vi "rsscope_core_global.vi"() -> ()   [LabVIEW 2014] (continued)
WfmRNOHist2, WfmTNTrack2, WfmDDNTrack2, WfmPNTrack2, WfmRNTrack2, WfmTNSpectrum2, WfmDDNSpectrum2, WfmPNSpectrum2, WfmRNSpectrum2, WfmPJDHist1, WfmBUJHist1, WfmRJHist1, WfmPJDTrack1, WfmPJDSpectrum1, WfmPJDHist2, WfmBUJHist2, WfmRJHist2, WfmPJDTrack2, WfmPJDSpectrum2, WfmPNDHist1, WfmBUNHist1, WfmRNHist1, WfmPNDTrack1, WfmPNDSpectrum1, WfmPNDHist2, WfmBUNHist2, WfmRNHist2, WfmPNDTrack2, WfmPNDSpectrum2\r\n\nRemote-control command(s):\nREFLevel<m>:AUTO:MODE"}, {"Level"=2, "Class Only"=FALSE, "Identifier"="RSSCOPE_ATTR_REFERENCE_LEVEL_AVERAGING_ENABLED", "Descriptive Name"="Reference Level Averaging Enabled", "Data Type"=3, "Command"="REFL{WfmSuffix}:AUTO", "Access"=2, "Range Table"="", "Read Callback"="", "Write Callback"="", "Supported Models"="", "Instrument Options"="", "Flags"=0, "Help"="Enables averaging over several histograms to determine the reference levels.\n\nAvailable Repeated Capabilities:\nWfmSuffix: WfmNone, WfmC1W1, WfmC1W2, WfmC1W3, WfmC2W1, WfmC2W2, WfmC2W3, WfmC3W1, WfmC3W2, WfmC3W3, WfmC4W1, WfmC4W2, WfmC4W3, WfmMath1, WfmMath2, WfmMath3, WfmMath4, WfmRef1, WfmRef2, WfmRef3, WfmRef4, WfmXY1, WfmXY2, WfmXY3, WfmXY4, WfmMeas1, WfmMeas2, WfmMeas3, WfmMeas4, WfmMeas5, WfmMeas6, WfmMeas7, WfmMeas8, WfmSbus1, WfmSbus2, WfmSbus3, WfmSbus4, WfmD0, WfmD1, WfmD2, WfmD3, WfmD4, WfmD5, WfmD6, WfmD7, WfmD8, WfmD9, WfmD10, WfmD11, WfmD12, WfmD13, WfmD14, WfmD15, WfmMSO1, WfmMSO2, WfmMSO3, WfmMSO4, WfmTRK1, WfmTRK2, WfmTRK3, WfmTRK4, WfmTRK5, WfmTRK6, WfmTRK7, WfmTRK8, WfmSpectrum1, WfmSpectrum2, WfmSpectrum3, WfmSpectrum4, WfmSG1TL1, WfmSG1TL2, WfmSG2TL1, WfmSG2TL2, WfmSG3TL1, WfmSG3TL2, WfmSG4TL1, WfmSG4TL2, WfmEye1, WfmEye2, WfmEye3, WfmEye4, WfmZ1V1, WfmZ1V2, WfmZ1V3, WfmZ1V4, WfmZ1I1, WfmZ1I2, WfmZ1I3, WfmZ1I4, WfmZ2V1, WfmZ2V2, WfmZ2V3, WfmZ2V4, WfmZ2I1, WfmZ2I2, WfmZ2I3, WfmZ2I4, WfmDiff1, WfmDiff2, WfmCommon1, WfmCommon2, WfmTDRZ, WfmTDRH, WfmTDRR, WfmMath5, WfmMath6, WfmMath7, WfmMath8, WfmSpectrum5, WfmSpectrum6, WfmSpectrum7, WfmSpectrum8, WfmSG5TL1, WfmSG5TL2, WfmSG6TL1, WfmSG6TL2, WfmSG7TL1, WfmSG7TL2, WfmSG8TL1, WfmSG8TL2, WfmHP1, WfmHP2, WfmHP3, WfmHP4, WfmHP5, WfmHP6, WfmHP7, WfmHP8, WfmHP9, WfmHP10, WfmBathtub1, WfmBathMeas1, WfmStepResp1, WfmSRHist1, WfmSDHist1, WfmTJHist1, WfmDJHist1, WfmDDJHist1, WfmPJHist1, WfmRJOHist1, WfmSRTrack1, WfmTJTrack1, WfmDJTrack1, WfmDDJTrack1, WfmPJTrack1, WfmRJTrack1, WfmTJSpectrum1, WfmDDJSpectrum1, WfmPJSpectrum1, WfmRJSpectrum1, WfmSEye1, WfmBathtub2, WfmBathMeas2, WfmStepResp2, WfmSRHist2, WfmSDHist2, WfmTJHist2, WfmDJHist2, WfmDDJHist2, WfmPJHist2, WfmRJOHist2, WfmSRTrack2, WfmSDTrack2, WfmTJTrack2, WfmDDJTrack2, WfmPJTrack2, WfmRJTrack2, WfmTJSpectrum2, WfmDDJSpectrum2, WfmPJSpectrum2, WfmRJSpectrum2, WfmSEye2, WfmNBathtub1, WfmNBathMeas1, WfmTNHist1, WfmDNHist1, WfmDDNHist1, WfmPNHist1, WfmRNOTrack1, WfmTNTrack1, WfmDDNTrack1, WfmPNTrack1, WfmRNTrack1, WfmTNSpectrum1, WfmDDNSpectrum1, WfmPNSpectrum1, WfmRNSpectrum1, WfmNBathtub2, WfmNBathMeas2, WfmTNHist2, WfmDNHist2, WfmDDNHist2, WfmPNHist2, WfmRNOHist2, WfmTNTrack2, WfmDDNTrack2, WfmPNTrack2, WfmRNTrack2, WfmTNSpectrum2, WfmDDNSpectrum2, WfmPNSpectrum2, WfmRNSpectrum2, WfmPJDHist1, WfmBUJHist1, WfmRJHist1, WfmPJDTrack1, WfmPJDSpectrum1, WfmPJDHist2, WfmBUJHist2, WfmRJHist2, WfmPJDTrack2, WfmPJDSpectrum2, WfmPNDHist1, WfmBUNHist1, WfmRNHist1, WfmPNDTrack1, WfmPNDSpectrum1, WfmPNDHist2, WfmBUNHist2, WfmRNHist2, WfmPNDTrack2, WfmPNDSpectrum2\r\n\nRemote-control command(s):\nREFLevel<m>:AUTO[:STATe]"}, {"Level"=2, "Class Only"=FALSE, "Identifier"="RSSCOPE_ATTR_REFERENCE_LEVEL_AVERAGING_COUNT", "Descriptive Name"="Reference Level Averaging Count", "Data Type"=0, "Command"="REFL{WfmSuffix}:AUTO:COUN", "Access"=2, "Range Table"="rsscope_rngRefLevelAvgCount", "Read Callback"="", "Write Callback"="", "Supported Models"="", "Instrument Options"="", "Flags"=0, "Help"="Defines the number of histograms to calculate the average from.\n\nAvailable Repeated Capabilities:\nWfmSuffix: WfmNone, WfmC1W1, WfmC1W2, WfmC1W3, WfmC2W1, WfmC2W2, WfmC2W3, WfmC3W1, WfmC3W2, WfmC3W3, WfmC4W1, WfmC4W2, WfmC4W3, WfmMath1, WfmMath2, WfmMath3, WfmMath4, WfmRef1, WfmRef2, WfmRef3, WfmRef4, WfmXY1, WfmXY2, WfmXY3, WfmXY4, WfmMeas1, WfmMeas2, WfmMeas3, WfmMeas4, WfmMeas5, WfmMeas6, WfmMeas7, WfmMeas8, WfmSbus1, WfmSbus2, WfmSbus3, WfmSbus4, WfmD0, WfmD1, WfmD2, WfmD3, WfmD4, WfmD5, WfmD6, WfmD7, WfmD8, WfmD9, WfmD10, WfmD11, WfmD12, WfmD13, WfmD14, WfmD15, WfmMSO1, WfmMSO2, WfmMSO3, WfmMSO4, WfmTRK1, WfmTRK2, WfmTRK3, WfmTRK4, WfmTRK5, WfmTRK6, WfmTRK7, WfmTRK8, WfmSpectrum1, WfmSpectrum2, WfmSpectrum3, WfmSpectrum4, WfmSG1TL1, WfmSG1TL2, WfmSG2TL1, WfmSG2TL2, WfmSG3TL1, WfmSG3TL2, WfmSG4TL1, WfmSG4TL2, WfmEye1, WfmEye2, WfmEye3, WfmEye4, WfmZ1V1, WfmZ1V2, WfmZ1V3, WfmZ1V4, WfmZ1I1, WfmZ1I2, WfmZ1I3, WfmZ1I4, WfmZ2V1, WfmZ2V2, WfmZ2V3, WfmZ2V4, WfmZ2I1, WfmZ2I2, WfmZ2I3, WfmZ2I4, WfmDiff1, WfmDiff2, WfmCommon1, WfmCommon2, WfmTDRZ, WfmTDRH, WfmTDRR, WfmMath5, WfmMath6, WfmMath7, WfmMath8, WfmSpectrum5, WfmSpectrum6, WfmSpectrum7, WfmSpectrum8, WfmSG5TL1, WfmSG5TL2, WfmSG6TL1, WfmSG6TL2, WfmSG7TL1, WfmSG7TL2, WfmSG8TL1, WfmSG8TL2, WfmHP1, WfmHP2, WfmHP3, WfmHP4, WfmHP5, WfmHP6, WfmHP7, WfmHP8, WfmHP9, WfmHP10, WfmBathtub1, WfmBathMeas1, WfmStepResp1, WfmSRHist1, WfmSDHist1, WfmTJHist1, WfmDJHist1, WfmDDJHist1, WfmPJHist1, WfmRJOHist1, WfmSRTrack1, WfmTJTrack1, WfmDJTrack1, WfmDDJTrack1, WfmPJTrack1, WfmRJTrack1, WfmTJSpectrum1, WfmDDJSpectrum1, WfmPJSpectrum1, WfmRJSpectrum1, WfmSEye1, WfmBathtub2, WfmBathMeas2, WfmStepResp2, WfmSRHist2, WfmSDHist2, WfmTJHist2, WfmDJHist2, WfmDDJHist2, WfmPJHist2, WfmRJOHist2, WfmSRTrack2, WfmSDTrack2, WfmTJTrack2, WfmDDJTrack2, WfmPJTrack2, WfmRJTrack2, WfmTJSpectrum2, WfmDDJSpectrum2, WfmPJSpectrum2, WfmRJSpectrum2, WfmSEye2, WfmNBathtub1, WfmNBathMeas1, WfmTNHist1, WfmDNHist1, WfmDDNHist1, WfmPNHist1, WfmRNOTrack1, WfmTNTrack1, WfmDDNTrack1, WfmPNTrack1, WfmRNTrack1, WfmTNSpectrum1, WfmDDNSpectrum1, WfmPNSpectrum1, WfmRNSpectrum1, WfmNBathtub2, WfmNBathMeas2, WfmTNHist2, WfmDNHist2, WfmDDNHist2, WfmPNHist2, WfmRNOHist2, WfmTNTrack2, WfmDDNTrack2, WfmPNTrack2, WfmRNTrack2, WfmTNSpectrum2, WfmDDNSpectrum2, WfmPNSpectrum2, WfmRNSpectrum2, WfmPJDHist1, WfmBUJHist1, WfmRJHist1, WfmPJDTrack1, WfmPJDSpectrum1, WfmPJDHist2, WfmBUJHist2, WfmRJHist2, WfmPJDTrack2, WfmPJDSpectrum2, WfmPNDHist1, WfmBUNHist1, WfmRNHist1, WfmPNDTrack1, WfmPNDSpectrum1, WfmPNDHist2, WfmBUNHist2, WfmRNHist2, WfmPNDTrack2, WfmPNDSpectrum2\r\n\nRemote-control command(s):\nREFLevel<m>:AUTO:COUNt"}, {"Level"=2, "Class Only"=TRUE, "Identifier"="", "Descriptive Name"="Reference User Signal Level", "Data Type"=0, "Command"="", "Access"=0, "Range Table"="", "Read Callback"="", "Write Callback"="", "Supported Models"="", "Instrument Options"="", "Flags"=0, "Help"="Contains reference level configuration for user signals."}, {"Level"=3, "Class Only"=FALSE, "Identifier"="RSSCOPE_ATTR_REFERENCE_USER_SIGNAL_HIGH", "Descriptive Name"="Reference User Signal High", "Data Type"=1, "Command"="REFL{WfmSuffix}:ABS:HIGH", "Access"=2, "Range Table"="", "Read Callback"="", "Write Callback"="", "Supported Models"="", "Instrument Options"="", "Flags"=0, "Help"="The signal value that represents a high level.\n\nAvailable Repeated Capabilities:\nWfmSuffix: WfmNone, WfmC1W1, WfmC1W2, WfmC1W3, WfmC2W1, WfmC2W2, WfmC2W3, WfmC3W1, WfmC3W2, WfmC3W3, WfmC4W1, WfmC4W2, WfmC4W3, WfmMath1, WfmMath2, WfmMath3, WfmMath4, WfmRef1, WfmRef2, WfmRef3, WfmRef4, WfmXY1, WfmXY2, WfmXY3, WfmXY4, WfmMeas1, WfmMeas2, WfmMeas3, WfmMeas4, WfmMeas5, WfmMeas6, WfmMeas7, WfmMeas8, WfmSbus1, WfmSbus2, WfmSbus3, WfmSbus4, WfmD0, WfmD1, WfmD2, WfmD3, WfmD4, WfmD5, WfmD6, WfmD7, WfmD8, WfmD9, WfmD10, WfmD11, WfmD12, WfmD13, WfmD14, WfmD15, WfmMSO1, WfmMSO2, WfmMSO3, WfmMSO4, WfmTRK1, WfmTRK2, WfmTRK3, WfmTRK4, WfmTRK5, WfmTRK6, WfmTRK7, WfmTRK8, WfmSpectrum1, WfmSpectrum2, WfmSpectrum3, WfmSpectrum4, WfmSG1TL1, WfmSG1TL2, WfmSG2TL1, WfmSG2TL2, WfmSG3TL1, WfmSG3TL2, WfmSG4TL1, WfmSG4TL2, WfmEye1, WfmEye2, WfmEye3, WfmEye4, WfmZ1V1, WfmZ1V2, WfmZ1V3, WfmZ1V4, WfmZ1I1, WfmZ1I2, WfmZ1I3, WfmZ1I4, WfmZ2V1, WfmZ2V2, WfmZ2V3, WfmZ2V4, WfmZ2I1, WfmZ2I2, WfmZ2I3, WfmZ2I4, WfmDiff1, WfmDiff2, WfmCommon1, WfmCommon2, WfmTDRZ, WfmTDRH, WfmTDRR, WfmMath5, WfmMath6, WfmMath7, WfmMath8, WfmSpectrum5, WfmSpectrum6, WfmSpectrum7, WfmSpectrum8, WfmSG5TL1, WfmSG5TL2, WfmSG6TL1, WfmSG6TL2, WfmSG7TL1, WfmSG7TL2, WfmSG8TL1, WfmSG8TL2, WfmHP1, WfmHP2, WfmHP3, WfmHP4, WfmHP5, WfmHP6, WfmHP7, WfmHP8, WfmHP9, WfmHP10, WfmBathtub1, WfmBathMeas1, WfmStepResp1, WfmSRHist1, WfmSDHist1, WfmTJHist1, WfmDJHist1, WfmDDJHist1, WfmPJHist1, WfmRJOHist1, WfmSRTrack1, WfmTJTrack1, WfmDJTrack1, WfmDDJTrack1, WfmPJTrack1, WfmRJTrack1, WfmTJSpectrum1, WfmDDJSpectrum1, WfmPJSpectrum1, WfmRJSpectrum1, WfmSEye1, WfmBathtub2, WfmBathMeas2, WfmStepResp2, WfmSRHist2, WfmSDHist2, WfmTJHist2, WfmDJHist2, WfmDDJHist2, WfmPJHist2, WfmRJOHist2, WfmSRTrack2, WfmSDTrack2, WfmTJTrack2, WfmDDJTrack2, WfmPJTrack2, WfmRJTrack2, WfmTJSpectrum2, WfmDDJSpectrum2, WfmPJSpectrum2, WfmRJSpectrum2, WfmSEye2, WfmNBathtub1, WfmNBathMeas1, WfmTNHist1, WfmDNHist1, WfmDDNHist1, WfmPNHist1, WfmRNOTrack1, WfmTNTrack1, WfmDDNTrack1, WfmPNTrack1, WfmRNTrack1, WfmTNSpectrum1, WfmDDNSpectrum1, WfmPNSpectrum1, WfmRNSpectrum1, WfmNBathtub2, WfmNBathMeas2, WfmTNHist2, WfmDNHist2, WfmDDNHist2, WfmPNHist2, WfmRNOHist2, WfmTNTrack2, WfmDDNTrack2, WfmPNTrack2, WfmRNTrack2, WfmTNSpectrum2, WfmDDNSpectrum2, WfmPNSpectrum2, WfmRNSpectrum2, WfmPJDHist1, WfmBUJHist1, WfmRJHist1, WfmPJDTrack1, WfmPJDSpectrum1, WfmPJDHist2, WfmBUJHist2, WfmRJHist2, WfmPJDTrack2, WfmPJDSpectrum2, WfmPNDHist1, WfmBUNHist1, WfmRNHist1, WfmPNDTrack1, WfmPNDSpectrum1, WfmPNDHist2, WfmBUNHist2, WfmRNHist2, WfmPNDTrack2, WfmPNDSpectrum2\r\n\nRemote-control command(s):\nREFLevel<m>:ABSolute:HIGH"}, {"Level"=3, "Class Only"=FALSE, "Identifier"="RSSCOPE_ATTR_REFERENCE_USER_SIGNAL_LOW", "Descriptive Name"="Reference User Signal Low", "Data Type"=1, "Command"="REFL{WfmSuffix}:ABS:LOW", "Access"=2, "Range Table"="", "Read Callback"="", "Write Callback"="", "Supported Models"="", "Instrument Options"="", "Flags"=0, "Help"="The signal value that represents a low level.\n\nAvailable Repeated Capabilities:\nWfmSuffix: WfmNone, WfmC1W1, WfmC1W2, WfmC1W3, WfmC2W1, WfmC2W2, WfmC2W3, WfmC3W1, WfmC3W2, WfmC3W3, WfmC4W1, WfmC4W2, WfmC4W3, WfmMath1, WfmMath2, WfmMath3, WfmMath4, WfmRef1, WfmRef2, WfmRef3, WfmRef4, WfmXY1, WfmXY2, WfmXY3, WfmXY4, WfmMeas1, WfmMeas2, WfmMeas3, WfmMeas4, WfmMeas5, WfmMeas6, WfmMeas7, WfmMeas8, WfmSbus1, WfmSbus2, WfmSbus3, WfmSbus4, WfmD0, WfmD1, WfmD2, WfmD3, WfmD4, WfmD5, WfmD6, WfmD7, WfmD8, WfmD9, WfmD10, WfmD11, WfmD12, WfmD13, WfmD14, WfmD15, WfmMSO1, WfmMSO2, WfmMSO3, WfmMSO4, WfmTRK1, WfmTRK2, WfmTRK3, WfmTRK4, WfmTRK5, WfmTRK6, WfmTRK7, WfmTRK8, WfmSpectrum1, WfmSpectrum2, WfmSpectrum3, WfmSpectrum4, WfmSG1TL1, WfmSG1TL2, WfmSG2TL1, WfmSG2TL2, WfmSG3TL1, WfmSG3TL2, WfmSG4TL1, WfmSG4TL2, WfmEye1, WfmEye2, WfmEye3, WfmEye4, WfmZ1V1, WfmZ1V2, WfmZ1V3, WfmZ1V4, WfmZ1I1, WfmZ1I2, WfmZ1I3, WfmZ1I4, WfmZ2V1, WfmZ2V2, WfmZ2V3, WfmZ2V4, WfmZ2I1, WfmZ2I2, WfmZ2I3, WfmZ2I4, WfmDiff1, WfmDiff2, WfmCommon1, WfmCommon2, WfmTDRZ, WfmTDRH, WfmTDRR, WfmMath5, WfmMath6, WfmMath7, WfmMath8, WfmSpectrum5, WfmSpectrum6, WfmSpectrum7, WfmSpectrum8, WfmSG5TL1, WfmSG5TL2, WfmSG6TL1, WfmSG6TL2, WfmSG7TL1, WfmSG7TL2, WfmSG8TL1, WfmSG8TL2, WfmHP1, WfmHP2, WfmHP3, WfmHP4, WfmHP5, WfmHP6, WfmHP7, WfmHP8, WfmHP9, WfmHP10, WfmBathtub1, WfmBathMeas1, WfmStepResp1, WfmSRHist1, WfmSDHist1, WfmTJHist1, WfmDJHist1, WfmDDJHist1, WfmPJHist1, WfmRJOHist1, WfmSRTrack1, WfmTJTrack1, WfmDJTrack1, WfmDDJTrack1, WfmPJTrack1, WfmRJTrack1, WfmTJSpectrum1, WfmDDJSpectrum1, WfmPJSpectrum1, WfmRJSpectrum1, WfmSEye1, WfmBathtub2, WfmBathMeas2, WfmStepResp2, WfmSRHist2, WfmSDHist2, WfmTJHist2, WfmDJHist2, WfmDDJHist2, WfmPJHist2, WfmRJOHist2, WfmSRTrack2, WfmSDTrack2, WfmTJTrack2, WfmDDJTrack2, WfmPJTrack2, WfmRJTrack2, WfmTJSpectrum2, WfmDDJSpectrum2, WfmPJSpectrum2, WfmRJSpectrum2, WfmSEye2, WfmNBathtub1, WfmNBathMeas1, WfmTNHist1, WfmDNHist1, WfmDDNHist1, WfmPNHist1, WfmRNOTrack1, WfmTNTrack1, WfmDDNTrack1, WfmPNTrack1, WfmRNTrack1, WfmTNSpectrum1, WfmDDNSpectrum1, WfmPNSpectrum1, WfmRNSpectrum1, WfmNBathtub2, WfmNBathMeas2, WfmTNHist2, WfmDNHist2, WfmDDNHist2, WfmPNHist2, WfmRNOHist2, WfmTNTrack2, WfmDDNTrack2, WfmPNTrack2, WfmRNTrack2, WfmTNSpectrum2, WfmDDNSpectrum2, WfmPNSpectrum2, WfmRNSpectrum2, WfmPJDHist1, WfmBUJHist1, WfmRJHist1, WfmPJDTrack1, WfmPJDSpectrum1, WfmPJDHist2, WfmBUJHist2, WfmRJHist2, WfmPJDTrack2, WfmPJDSpectrum2, WfmPNDHist1, WfmBUNHist1, WfmRNHist1, WfmPNDTrack1, WfmPNDSpectrum1, WfmPNDHist2, WfmBUNHist2, WfmRNHist2, WfmPNDTrack2, WfmPNDSpectrum2\r\n\nRemote-control command(s):\nREFLevel<m>:ABSolute:LOW"}, {"Level"=3, "Class Only"=FALSE, "Identifier"="RSSCOPE_ATTR_REFERENCE_USER_TOP_DISTANCE", "Descriptive Name"="Reference User Top Distance", "Data Type"=1, "Command"="REFL{WfmSuffix}:ABS:TDIS", "Access"=2, "Range Table"="", "Read Callback"="", "Write Callback"="", "Supported Models"="", "Instrument Options"="", "Flags"=0, "Help"="The distance between the high signal level and the upper reference level.\n\nAvailable Repeated Capabilities:\nWfmSuffix: WfmNone, WfmC1W1, WfmC1W2, WfmC1W3, WfmC2W1, WfmC2W2, WfmC2W3, WfmC3W1, WfmC3W2, WfmC3W3, WfmC4W1, WfmC4W2, WfmC4W3, WfmMath1, WfmMath2, WfmMath3, WfmMath4, WfmRef1, WfmRef2, WfmRef3, WfmRef4, WfmXY1, WfmXY2, WfmXY3, WfmXY4, WfmMeas1, WfmMeas2, WfmMeas3, WfmMeas4, WfmMeas5, WfmMeas6, WfmMeas7, WfmMeas8, WfmSbus1, WfmSbus2, WfmSbus3, WfmSbus4, WfmD0, WfmD1, WfmD2, WfmD3, WfmD4, WfmD5, WfmD6, WfmD7, WfmD8, WfmD9, WfmD10, WfmD11, WfmD12, WfmD13, WfmD14, WfmD15, WfmMSO1, WfmMSO2, WfmMSO3, WfmMSO4, WfmTRK1, WfmTRK2, WfmTRK3, WfmTRK4, WfmTRK5, WfmTRK6, WfmTRK7, WfmTRK8, WfmSpectrum1, WfmSpectrum2, WfmSpectrum3, WfmSpectrum4, WfmSG1TL1, WfmSG1TL2, WfmSG2TL1, WfmSG2TL2, WfmSG3TL1, WfmSG3TL2, WfmSG4TL1, WfmSG4TL2, WfmEye1, WfmEye2, WfmEye3, WfmEye4, WfmZ1V1, WfmZ1V2, WfmZ1V3, WfmZ1V4, WfmZ1I1, WfmZ1I2, WfmZ1I3, WfmZ1I4, WfmZ2V1, WfmZ2V2, WfmZ2V3, WfmZ2V4, WfmZ2I1, WfmZ2I2, WfmZ2I3, WfmZ2I4, WfmDiff1, WfmDiff2, WfmCommon1, WfmCommon2, WfmTDRZ, WfmTDRH, WfmTDRR, WfmMath5, WfmMath6, WfmMath7, WfmMath8, WfmSpectrum5, WfmSpectrum6, WfmSpectrum7, WfmSpectrum8, WfmSG5TL1, WfmSG5TL2, WfmSG6TL1, WfmSG6TL2, WfmSG7TL1, WfmSG7TL2, WfmSG8TL1, WfmSG8TL2, WfmHP1, WfmHP2, WfmHP3, WfmHP4, WfmHP5, WfmHP6, WfmHP7, WfmHP8, WfmHP9, WfmHP10, WfmBathtub1, WfmBathMeas1, WfmStepResp1, WfmSRHist1, WfmSDHist1, WfmTJHist1, WfmDJHist1, WfmDDJHist1, WfmPJHist1, WfmRJOHist1, WfmSRTrack1, WfmTJTrack1, WfmDJTrack1, WfmDDJTrack1, WfmPJTrack1, WfmRJTrack1, WfmTJSpectrum1, WfmDDJSpectrum1, WfmPJSpectrum1, WfmRJSpectrum1, WfmSEye1, WfmBathtub2, WfmBathMeas2, WfmStepResp2, WfmSRHist2, WfmSDHist2, WfmTJHist2, WfmDJHist2, WfmDDJHist2, WfmPJHist2, WfmRJOHist2, WfmSRTrack2, WfmSDTrack2, WfmTJTrack2, WfmDDJTrack2, WfmPJTrack2, WfmRJTrack2, WfmTJSpectrum2, WfmDDJSpectrum2, WfmPJSpectrum2, WfmRJSpectrum2, WfmSEye2, WfmNBathtub1, WfmNBathMeas1, WfmTNHist1, WfmDNHist1, WfmDDNHist1, WfmPNHist1, WfmRNOTrack1, WfmTNTrack1, WfmDDNTrack1, WfmPNTrack1, WfmRNTrack1, WfmTNSpectrum1, WfmDDNSpectrum1, WfmPNSpectrum1, WfmRNSpectrum1, WfmNBathtub2, WfmNBathMeas2, WfmTNHist2, WfmDNHist2, WfmDDNHist2, WfmPNHist2, WfmRNOHist2, WfmTNTrack2, WfmDDNTrack2, WfmPNTrack2, WfmRNTrack2, WfmTNSpectrum2, WfmDDNSpectrum2, WfmPNSpectrum2, WfmRNSpectrum2, WfmPJDHist1, WfmBUJHist1, WfmRJHist1, WfmPJDTrack1, WfmPJDSpectrum1, WfmPJDHist2, WfmBUJHist2, WfmRJHist2, WfmPJDTrack2, WfmPJDSpectrum2, WfmPNDHist1, WfmBUNHist1, WfmRNHist1, WfmPNDTrack1, WfmPNDSpectrum1, WfmPNDHist2, WfmBUNHist2, WfmRNHist2, WfmPNDTrack2, WfmPNDSpectrum2\r\n\nRemote-control command(s):\nREFLevel<m>:ABSolute:TDIStance"}, {"Level"=3, "Class Only"=FALSE, "Identifier"="RSSCOPE_ATTR_REFERENCE_USER_BOTTOM_DISTANCE", "Descriptive Name"="Reference User Bottom Distance", "Data Type"=1, "Command"="REFL{WfmSuffix}:ABS:BDIS", "Access"=2, "Range Table"="", "Read Callback"="", "Write Callback"="", "Supported Models"="", "Instrument Options"="", "Flags"=0, "Help"="The distance between the lower reference level and the low signal value.\n\nAvailable Repeated Capabilities:\nWfmSuffix: WfmNone, WfmC1W1, WfmC1W2, WfmC1W3, WfmC2W1, WfmC2W2, WfmC2W3, WfmC3W1, WfmC3W2, WfmC3W3, WfmC4W1, WfmC4W2, WfmC4W3, WfmMath1, WfmMath2, WfmMath3, WfmMath4, WfmRef1, WfmRef2, WfmRef3, WfmRef4, WfmXY1, WfmXY2, WfmXY3, WfmXY4, WfmMeas1, WfmMeas2, WfmMeas3, WfmMeas4, WfmMeas5, WfmMeas6, WfmMeas7, WfmMeas8, WfmSbus1, WfmSbus2, WfmSbus3, WfmSbus4, WfmD0, WfmD1, WfmD2, WfmD3, WfmD4, WfmD5, WfmD6, WfmD7, WfmD8, WfmD9, WfmD10, WfmD11, WfmD12, WfmD13, WfmD14, WfmD15, WfmMSO1, WfmMSO2, WfmMSO3, WfmMSO4, WfmTRK1, WfmTRK2, WfmTRK3, WfmTRK4, WfmTRK5, WfmTRK6, WfmTRK7, WfmTRK8, WfmSpectrum1, WfmSpectrum2, WfmSpectrum3, WfmSpectrum4, WfmSG1TL1, WfmSG1TL2, WfmSG2TL1, WfmSG2TL2, WfmSG3TL1, WfmSG3TL2, WfmSG4TL1, WfmSG4TL2, WfmEye1, WfmEye2, WfmEye3, WfmEye4, WfmZ1V1, WfmZ1V2, WfmZ1V3, WfmZ1V4, WfmZ1I1, WfmZ1I2, WfmZ1I3, WfmZ1I4, WfmZ2V1, WfmZ2V2, WfmZ2V3, WfmZ2V4, WfmZ2I1, WfmZ2I2, WfmZ2I3, WfmZ2I4, WfmDiff1, WfmDiff2, WfmCommon1, WfmCommon2, WfmTDRZ, WfmTDRH, WfmTDRR, WfmMath5, WfmMath6, WfmMath7, WfmMath8, WfmSpectrum5, WfmSpectrum6, WfmSpectrum7, WfmSpectrum8, WfmSG5TL1, WfmSG5TL2, WfmSG6TL1, WfmSG6TL2, WfmSG7TL1, WfmSG7TL2, WfmSG8TL1, WfmSG8TL2, WfmHP1, WfmHP2, WfmHP3, WfmHP4, WfmHP5, WfmHP6, WfmHP7, WfmHP8, WfmHP9, WfmHP10, WfmBathtub1, WfmBathMeas1, WfmStepResp1, WfmSRHist1, WfmSDHist1, WfmTJHist1, WfmDJHist1, WfmDDJHist1, WfmPJHist1, WfmRJOHist1, WfmSRTrack1, WfmTJTrack1, WfmDJTrack1, WfmDDJTrack1, WfmPJTrack1, WfmRJTrack1, WfmTJSpectrum1, WfmDDJSpectrum1, WfmPJSpectrum1, WfmRJSpectrum1, WfmSEye1, WfmBathtub2, WfmBathMeas2, WfmStepResp2, WfmSRHist2, WfmSDHist2, WfmTJHist2, WfmDJHist2, WfmDDJHist2, WfmPJHist2, WfmRJOHist2, WfmSRTrack2, WfmSDTrack2, WfmTJTrack2, WfmDDJTrack2, WfmPJTrack2, WfmRJTrack2, WfmTJSpectrum2, WfmDDJSpectrum2, WfmPJSpectrum2, WfmRJSpectrum2, WfmSEye2, WfmNBathtub1, WfmNBathMeas1, WfmTNHist1, WfmDNHist1, WfmDDNHist1, WfmPNHist1, WfmRNOTrack1, WfmTNTrack1, WfmDDNTrack1, WfmPNTrack1, WfmRNTrack1, WfmTNSpectrum1, WfmDDNSpectrum1, WfmPNSpectrum1, WfmRNSpectrum1, WfmNBathtub2, WfmNBathMeas2, WfmTNHist2, WfmDNHist2, WfmDDNHist2, WfmPNHist2, WfmRNOHist2, WfmTNTrack2, WfmDDNTrack2, WfmPNTrack2, WfmRNTrack2, WfmTNSpectrum2, WfmDDNSpectrum2, WfmPNSpectrum2, WfmRNSpectrum2, WfmPJDHist1, WfmBUJHist1, WfmRJHist1, WfmPJDTrack1, WfmPJDSpectrum1, WfmPJDHist2, WfmBUJHist2, WfmRJHist2, WfmPJDTrack2, WfmPJDSpectrum2, WfmPNDHist1, WfmBUNHist1, WfmRNHist1, WfmPNDTrack1, WfmPNDSpectrum1, WfmPNDHist2, WfmBUNHist2, WfmRNHist2, WfmPNDTrack2, WfmPNDSpectrum2\r\n\nRemote-control command(s):\nREFLevel<m>:ABSolute:BDIStance"}, {"Level"=2, "Class Only"=TRUE, "Identifier"="", "Descriptive Name"="User Reference Level", "Data Type"=0, "Command"="", "Access"=0, "Range Table"="", "Read Callback"="", "Write Callback"="", "Supported Models"="", "Instrument Options"="", "Flags"=0, "Help"="Contains user reference level configuration."}, {"Level"=3, "Class Only"=FALSE, "Identifier"="RSSCOPE_ATTR_USER_REFERENCE_UPPER_LEVEL", "Descriptive Name"="User Reference Upper Level", "Data Type"=1, "Command"="REFL{WfmSuffix}:ABS:ULEV", "Access"=2, "Range Table"="", "Read Callback"="", "Write Callback"="", "Supported Models"="", "Instrument Options"="", "Flags"=0, "Help"="The upper reference level, required e.g. to determine a rise.\n\nAvailable Repeated Capabilities:\nWfmSuffix: WfmNone, WfmC1W1, WfmC1W2, WfmC1W3, WfmC2W1, WfmC2W2, WfmC2W3, WfmC3W1, WfmC3W2, WfmC3W3, WfmC4W1, WfmC4W2, WfmC4W3, WfmMath1, WfmMath2, WfmMath3, WfmMath4, WfmRef1, WfmRef2, WfmRef3, WfmRef4, WfmXY1, WfmXY2, WfmXY3, WfmXY4, WfmMeas1, WfmMeas2, WfmMeas3, WfmMeas4, WfmMeas5, WfmMeas6, WfmMeas7, WfmMeas8, WfmSbus1, WfmSbus2, WfmSbus3, WfmSbus4, WfmD0, WfmD1, WfmD2, WfmD3, WfmD4, WfmD5, WfmD6, WfmD7, WfmD8, WfmD9, WfmD10, WfmD11, WfmD12, WfmD13, WfmD14, WfmD15, WfmMSO1, WfmMSO2, WfmMSO3, WfmMSO4, WfmTRK1, WfmTRK2, WfmTRK3, WfmTRK4, WfmTRK5, WfmTRK6, WfmTRK7, WfmTRK8, WfmSpectrum1, WfmSpectrum2, WfmSpectrum3, WfmSpectrum4, WfmSG1TL1, WfmSG1TL2, WfmSG2TL1, WfmSG2TL2, WfmSG3TL1, WfmSG3TL2, WfmSG4TL1, WfmSG4TL2, WfmEye1, WfmEye2, WfmEye3, WfmEye4, WfmZ1V1, WfmZ1V2, WfmZ1V3, WfmZ1V4, WfmZ1I1, WfmZ1I2, WfmZ1I3, WfmZ1I4, WfmZ2V1, WfmZ2V2, WfmZ2V3, WfmZ2V4, WfmZ2I1, WfmZ2I2, WfmZ2I3, WfmZ2I4, WfmDiff1, WfmDiff2, WfmCommon1, WfmCommon2, WfmTDRZ, WfmTDRH, WfmTDRR, WfmMath5, WfmMath6, WfmMath7, WfmMath8, WfmSpectrum5, WfmSpectrum6, WfmSpectrum7, WfmSpectrum8, WfmSG5TL1, WfmSG5TL2, WfmSG6TL1, WfmSG6TL2, WfmSG7TL1, WfmSG7TL2, WfmSG8TL1, WfmSG8TL2, WfmHP1, WfmHP2, WfmHP3, WfmHP4, WfmHP5, WfmHP6, WfmHP7, WfmHP8, WfmHP9, WfmHP10, WfmBathtub1, WfmBathMeas1, WfmStepResp1, WfmSRHist1, WfmSDHist1, WfmTJHist1, WfmDJHist1, WfmDDJHist1, WfmPJHist1, WfmRJOHist1, WfmSRTrack1, WfmTJTrack1, WfmDJTrack1, WfmDDJTrack1, WfmPJTrack1, WfmRJTrack1, WfmTJSpectrum1, WfmDDJSpectrum1, WfmPJSpectrum1, WfmRJSpectrum1, WfmSEye1, WfmBathtub2, WfmBathMeas2, WfmStepResp2, WfmSRHist2, WfmSDHist2, WfmTJHist2, WfmDJHist2, WfmDDJHist2, WfmPJHist2, WfmRJOHist2, WfmSRTrack2, WfmSDTrack2, WfmTJTrack2, WfmDDJTrack2, WfmPJTrack2, WfmRJTrack2, WfmTJSpectrum2, WfmDDJSpectrum2, WfmPJSpectrum2, WfmRJSpectrum2, WfmSEye2, WfmNBathtub1, WfmNBathMeas1, WfmTNHist1, WfmDNHist1, WfmDDNHist1, WfmPNHist1, WfmRNOTrack1, WfmTNTrack1, WfmDDNTrack1, WfmPNTrack1, WfmRNTrack1, WfmTNSpectrum1, WfmDDNSpectrum1, WfmPNSpectrum1, WfmRNSpectrum1, WfmNBathtub2, WfmNBathMeas2, WfmTNHist2, WfmDNHist2, WfmDDNHist2, WfmPNHist2, WfmRNOHist2, WfmTNTrack2, WfmDDNTrack2, WfmPNTrack2, WfmRNTrack2, WfmTNSpectrum2, WfmDDNSpectrum2, WfmPNSpectrum2, WfmRNSpectrum2, WfmPJDHist1, WfmBUJHist1, WfmRJHist1, WfmPJDTrack1, WfmPJDSpectrum1, WfmPJDHist2, WfmBUJHist2, WfmRJHist2, WfmPJDTrack2, WfmPJDSpectrum2, WfmPNDHist1, WfmBUNHist1, WfmRNHist1, WfmPNDTrack1, WfmPNDSpectrum1, WfmPNDHist2, WfmBUNHist2, WfmRNHist2, WfmPNDTrack2, WfmPNDSpectrum2\r\n\nRemote-control command(s):\nREFLevel<m>:ABSolute:ULEVel"}, {"Level"=3, "Class Only"=FALSE, "Identifier"="RSSCOPE_ATTR_USER_REFERENCE_LOWER_LEVEL", "Descriptive Name"="User Reference Lower Level", "Data Type"=1, "Command"="REFL{WfmSuffix}:ABS:LLEV", "Access"=2, "Range Table"="", "Read Callback"="", "Write Callback"="", "Supported Models"="", "Instrument Options"="", "Flags"=0, "Help"="The lower reference level, required e.g. to determine a fall.\n\nAvailable Repeated Capabilities:\nWfmSuffix: WfmNone, WfmC1W1, WfmC1W2, WfmC1W3, WfmC2W1, WfmC2W2, WfmC2W3, WfmC3W1, WfmC3W2, WfmC3W3, WfmC4W1, WfmC4W2, WfmC4W3, WfmMath1, WfmMath2, WfmMath3, WfmMath4, WfmRef1, WfmRef2, WfmRef3, WfmRef4, WfmXY1, WfmXY2, WfmXY3, WfmXY4, WfmMeas1, WfmMeas2, WfmMeas3, WfmMeas4, WfmMeas5, WfmMeas6, WfmMeas7, WfmMeas8, WfmSbus1, WfmSbus2, WfmSbus3, WfmSbus4, WfmD0, WfmD1, WfmD2, WfmD3, WfmD4, WfmD5, WfmD6, WfmD7, WfmD8, WfmD9, WfmD10, WfmD11, WfmD12, WfmD13, WfmD14, WfmD15, WfmMSO1, WfmMSO2, WfmMSO3, WfmMSO4, WfmTRK1, WfmTRK2, WfmTRK3, WfmTRK4, WfmTRK5, WfmTRK6, WfmTRK7, WfmTRK8, WfmSpectrum1, WfmSpectrum2, WfmSpectrum3, WfmSpectrum4, WfmSG1TL1, WfmSG1TL2, WfmSG2TL1, WfmSG2TL2, WfmSG3TL1, WfmSG3TL2, WfmSG4TL1, WfmSG4TL2, WfmEye1, WfmEye2, WfmEye3, WfmEye4, WfmZ1V1, WfmZ1V2, WfmZ1V3, WfmZ1V4, WfmZ1I1, WfmZ1I2, WfmZ1I3, WfmZ1I4, WfmZ2V1, WfmZ2V2, WfmZ2V3, WfmZ2V4, WfmZ2I1, WfmZ2I2, WfmZ2I3, WfmZ2I4, WfmDiff1, WfmDiff2, WfmCommon1, WfmCommon2, WfmTDRZ, WfmTDRH, WfmTDRR, WfmMath5, WfmMath6, WfmMath7, WfmMath8, WfmSpectrum5, WfmSpectrum6, WfmSpectrum7, WfmSpectrum8, WfmSG5TL1, WfmSG5TL2, WfmSG6TL1, WfmSG6TL2, WfmSG7TL1, WfmSG7TL2, WfmSG8TL1, WfmSG8TL2, WfmHP1, WfmHP2, WfmHP3, WfmHP4, WfmHP5, WfmHP6, WfmHP7, WfmHP8, WfmHP9, WfmHP10, WfmBathtub1, WfmBathMeas1, WfmStepResp1, WfmSRHist1, WfmSDHist1, WfmTJHist1, WfmDJHist1, WfmDDJHist1, WfmPJHist1, WfmRJOHist1, WfmSRTrack1, WfmTJTrack1, WfmDJTrack1, WfmDDJTrack1, WfmPJTrack1, WfmRJTrack1, WfmTJSpectrum1, WfmDDJSpectrum1, WfmPJSpectrum1, WfmRJSpectrum1, WfmSEye1, WfmBathtub2, WfmBathMeas2, WfmStepResp2, WfmSRHist2, WfmSDHist2, WfmTJHist2, WfmDJHist2, WfmDDJHist2, WfmPJHist2, WfmRJOHist2, WfmSRTrack2, WfmSDTrack2, WfmTJTrack2, WfmDDJTrack2, WfmPJTrack2, WfmRJTrack2, WfmTJSpectrum2, WfmDDJSpectrum2, WfmPJSpectrum2, WfmRJSpectrum2, WfmSEye2, WfmNBathtub1, WfmNBathMeas1, WfmTNHist1, WfmDNHist1, WfmDDNHist1, WfmPNHist1, WfmRNOTrack1, WfmTNTrack1, WfmDDNTrack1, WfmPNTrack1, WfmRNTrack1, WfmTNSpectrum1, WfmDDNSpectrum1, WfmPNSpectrum1, WfmRNSpectrum1, WfmNBathtub2, WfmNBathMeas2, WfmTNHist2, WfmDNHist2, WfmDDNHist2, WfmPNHist2, WfmRNOHist2, WfmTNTrack2, WfmDDNTrack2, WfmPNTrack2, WfmRNTrack2, WfmTNSpectrum2, WfmDDNSpectrum2, WfmPNSpectrum2, WfmRNSpectrum2, WfmPJDHist1, WfmBUJHist1, WfmRJHist1, WfmPJDTrack1, WfmPJDSpectrum1, WfmPJDHist2, WfmBUJHist2, WfmRJHist2, WfmPJDTrack2, WfmPJDSpectrum2, WfmPNDHist1, WfmBUNHist1, WfmRNHist1, WfmPNDTrack1, WfmPNDSpectrum1, WfmPNDHist2, WfmBUNHist2, WfmRNHist2, WfmPNDTrack2, WfmPNDSpectrum2\r\n\nRemote-control command(s):\nREFLevel<m>:ABSolute:LLEVel"}, {"Level"=3, "Class Only"=FALSE, "Identifier"="RSSCOPE_ATTR_USER_REFERENCE_MIDDLE_LEVEL", "Descriptive Name"="User Reference Middle Level", "Data Type"=1, "Command"="REFL{WfmSuffix}:ABS:MLEV", "Access"=2, "Range Table"="", "Read Callback"="", "Write Callback"="", "Supported Models"="", "Instrument Options"="", "Flags"=0, "Help"="The middle reference level.\n\nAvailable Repeated Capabilities:\nWfmSuffix: WfmNone, WfmC1W1, WfmC1W2, WfmC1W3, WfmC2W1, WfmC2W2, WfmC2W3, WfmC3W1, WfmC3W2, WfmC3W3, WfmC4W1, WfmC4W2, WfmC4W3, WfmMath1, WfmMath2, WfmMath3, WfmMath4, WfmRef1, WfmRef2, WfmRef3, WfmRef4, WfmXY1, WfmXY2, WfmXY3, WfmXY4, WfmMeas1, WfmMeas2, WfmMeas3, WfmMeas4, WfmMeas5, WfmMeas6, WfmMeas7, WfmMeas8, WfmSbus1, WfmSbus2, WfmSbus3, WfmSbus4, WfmD0, WfmD1, WfmD2, WfmD3, WfmD4, WfmD5, WfmD6, WfmD7, WfmD8, WfmD9, WfmD10, WfmD11, WfmD12, WfmD13, WfmD14, WfmD15, WfmMSO1, WfmMSO2, WfmMSO3, WfmMSO4, WfmTRK1, WfmTRK2, WfmTRK3, WfmTRK4, WfmTRK5, WfmTRK6, WfmTRK7, WfmTRK8, WfmSpectrum1, WfmSpectrum2, WfmSpectrum3, WfmSpectrum4, WfmSG1TL1, WfmSG1TL2, WfmSG2TL1, WfmSG2TL2, WfmSG3TL1, WfmSG3TL2, WfmSG4TL1, WfmSG4TL2, WfmEye1, WfmEye2, WfmEye3, WfmEye4, WfmZ1V1, WfmZ1V2, WfmZ1V3, WfmZ1V4, WfmZ1I1, WfmZ1I2, WfmZ1I3, WfmZ1I4, WfmZ2V1, WfmZ2V2, WfmZ2V3, WfmZ2V4, WfmZ2I1, WfmZ2I2, WfmZ2I3, WfmZ2I4, WfmDiff1, WfmDiff2, WfmCommon1, WfmCommon2, WfmTDRZ, WfmTDRH, WfmTDRR, WfmMath5, WfmMath6, WfmMath7, WfmMath8, WfmSpectrum5, WfmSpectrum6, WfmSpectrum7, WfmSpectrum8, WfmSG5TL1, WfmSG5TL2, WfmSG6TL1, WfmSG6TL2, WfmSG7TL1, WfmSG7TL2, WfmSG8TL1, WfmSG8TL2, WfmHP1, WfmHP2, WfmHP3, WfmHP4, WfmHP5, WfmHP6, WfmHP7, WfmHP8, WfmHP9, WfmHP10, WfmBathtub1, WfmBathMeas1, WfmStepResp1, WfmSRHist1, WfmSDHist1, WfmTJHist1, WfmDJHist1, WfmDDJHist1, WfmPJHist1, WfmRJOHist1, WfmSRTrack1, WfmTJTrack1, WfmDJTrack1, WfmDDJTrack1, WfmPJTrack1, WfmRJTrack1, WfmTJSpectrum1, WfmDDJSpectrum1, WfmPJSpectrum1, WfmRJSpectrum1, WfmSEye1, WfmBathtub2, WfmBathMeas2, WfmStepResp2, WfmSRHist2, WfmSDHist2, WfmTJHist2, WfmDJHist2, WfmDDJHist2, WfmPJHist2, WfmRJOHist2, WfmSRTrack2, WfmSDTrack2, WfmTJTrack2, WfmDDJTrack2, WfmPJTrack2, WfmRJTrack2, WfmTJSpectrum2, WfmDDJSpectrum2, WfmPJSpectrum2, WfmRJSpectrum2, WfmSEye2, WfmNBathtub1, WfmNBathMeas1, WfmTNHist1, WfmDNHist1, WfmDDNHist1, WfmPNHist1, WfmRNOTrack1, WfmTNTrack1, WfmDDNTrack1, WfmPNTrack1, WfmRNTrack1, WfmTNSpectrum1, WfmDDNSpectrum1, WfmPNSpectrum1, WfmRNSpectrum1, WfmNBathtub2, WfmNBathMeas2, WfmTNHist2, WfmDNHist2, WfmDDNHist2, WfmPNHist2, WfmRNOHist2, WfmTNTrack2, WfmDDNTrack2, WfmPNTrack2, WfmRNTrack2, WfmTNSpectrum2, WfmDDNSpectrum2, WfmPNSpectrum2, WfmRNSpectrum2, WfmPJDHist1, WfmBUJHist1, WfmRJHist1, WfmPJDTrack1, WfmPJDSpectrum1, WfmPJDHist2, WfmBUJHist2, WfmRJHist2, WfmPJDTrack2, WfmPJDSpectrum2, WfmPNDHist1, WfmBUNHist1, WfmRNHist1, WfmPNDTrack1, WfmPNDSpectrum1, WfmPNDHist2, WfmBUNHist2, WfmRNHist2, WfmPNDTrack2, WfmPNDSpectrum2\r\n\nRemote-control command(s):\nREFLevel<m>:ABSolute:MLEVel"}, {"Level"=3, "Class Only"=FALSE, "Identifier"="RSSCOPE_ATTR_USER_REFERENCE_RELATIVE_UPPER_LEVEL", "Descriptive Name"="User Reference Relative Upper Level", "Data Type"=0, "Command"="REFL{WfmSuffix}:REL:UPP", "Access"=2, "Range Table"="RsScope_rngUserReferenceRelativeLevel", "Read Callback"="", "Write Callback"="", "Supported Models"="", "Instrument Options"="", "Flags"=0, "Help"="Sets the upper  relative reference level, defined as a percentage of the high signal level.\n\nNote:\nRequires RSSCOPE_ATTR_REFERENCE_LEVEL_RELATIVE_LEVELS to be set to USER.\n\nAvailable Repeated Capabilities:\nWfmSuffix: WfmNone, WfmC1W1, WfmC1W2, WfmC1W3, WfmC2W1, WfmC2W2, WfmC2W3, WfmC3W1, WfmC3W2, WfmC3W3, WfmC4W1, WfmC4W2, WfmC4W3, WfmMath1, WfmMath2, WfmMath3, WfmMath4, WfmRef1, WfmRef2, WfmRef3, WfmRef4, WfmXY1, WfmXY2, WfmXY3, WfmXY4, WfmMeas1, WfmMeas2, WfmMeas3, WfmMeas4, WfmMeas5, WfmMeas6, WfmMeas7, WfmMeas8, WfmSbus1, WfmSbus2, WfmSbus3, WfmSbus4, WfmD0, WfmD1, WfmD2, WfmD3, WfmD4, WfmD5, WfmD6, WfmD7, WfmD8, WfmD9, WfmD10, WfmD11, WfmD12, WfmD13, WfmD14, WfmD15, WfmMSO1, WfmMSO2, WfmMSO3, WfmMSO4, WfmTRK1, WfmTRK2, WfmTRK3, WfmTRK4, WfmTRK5, WfmTRK6, WfmTRK7, WfmTRK8, WfmSpectrum1, WfmSpectrum2, WfmSpectrum3, WfmSpectrum4, WfmSG1TL1, WfmSG1TL2, WfmSG2TL1, WfmSG2TL2, WfmSG3TL1, WfmSG3TL2, WfmSG4TL1, WfmSG4TL2, WfmEye1, WfmEye2, WfmEye3, WfmEye4, WfmZ1V1, WfmZ1V2, WfmZ1V3, WfmZ1V4, WfmZ1I1, WfmZ1I2, WfmZ1I3, WfmZ1I4, WfmZ2V1, WfmZ2V2, WfmZ2V3, WfmZ2V4, WfmZ2I1, WfmZ2I2, WfmZ2I3, WfmZ2I4, WfmDiff1, WfmDiff2, WfmCommon1, WfmCommon2, WfmTDRZ, WfmTDRH, WfmTDRR, WfmMath5, WfmMath6, WfmMath7, WfmMath8, WfmSpectrum5, WfmSpectrum6, WfmSpectrum7, WfmSpectrum8, WfmSG5TL1, WfmSG5TL2, WfmSG6TL1, WfmSG6TL2, WfmSG7TL1, WfmSG7TL2, WfmSG8TL1, WfmSG8TL2, WfmHP1, WfmHP2, WfmHP3, WfmHP4, WfmHP5, WfmHP6, WfmHP7, WfmHP8, WfmHP9, WfmHP10, WfmBathtub1, WfmBathMeas1, WfmStepResp1, WfmSRHist1, WfmSDHist1, WfmTJHist1, WfmDJHist1, WfmDDJHist1, WfmPJHist1, WfmRJOHist1, WfmSRTrack1, WfmTJTrack1, WfmDJTrack1, WfmDDJTrack1, WfmPJTrack1, WfmRJTrack1, WfmTJSpectrum1, WfmDDJSpectrum1, WfmPJSpectrum1, WfmRJSpectrum1, WfmSEye1, WfmBathtub2, WfmBathMeas2, WfmStepResp2, WfmSRHist2, WfmSDHist2, WfmTJHist2, WfmDJHist2, WfmDDJHist2, WfmPJHist2, WfmRJOHist2, WfmSRTrack2, WfmSDTrack2, WfmTJTrack2, WfmDDJTrack2, WfmPJTrack2, WfmRJTrack2, WfmTJSpectrum2, WfmDDJSpectrum2, WfmPJSpectrum2, WfmRJSpectrum2, WfmSEye2, WfmNBathtub1, WfmNBathMeas1, WfmTNHist1, WfmDNHist1, WfmDDNHist1, WfmPNHist1, WfmRNOTrack1, WfmTNTrack1, WfmDDNTrack1, WfmPNTrack1, WfmRNTrack1, WfmTNSpectrum1, WfmDDNSpectrum1, WfmPNSpectrum1, WfmRNSpectrum1, WfmNBathtub2, WfmNBathMeas2, WfmTNHist2, WfmDNHist2, WfmDDNHist2, WfmPNHist2, WfmRNOHist2, WfmTNTrack2, WfmDDNTrack2, WfmPNTrack2, WfmRNTrack2, WfmTNSpectrum2, WfmDDNSpectrum2, WfmPNSpectrum2, WfmRNSpectrum2, WfmPJDHist1, WfmBUJHist1, WfmRJHist1, WfmPJDTrack1, WfmPJDSpectrum1, WfmPJDHist2, WfmBUJHist2, WfmRJHist2, WfmPJDTrack2, WfmPJDSpectrum2, WfmPNDHist1, WfmBUNHist1, WfmRNHist1, WfmPNDTrack1, WfmPNDSpectrum1, WfmPNDHist2, WfmBUNHist2, WfmRNHist2, WfmPNDTrack2, WfmPNDSpectrum2\r\n\nRemote-control command(s):\nREFLevel<m>:RELative:UPPer"}, {"Level"=3, "Class Only"=FALSE, "Identifier"="RSSCOPE_ATTR_USER_REFERENCE_RELATIVE_MIDDLE_LEVEL", "Descriptive Name"="User Reference Relative Middle Level", "Data Type"=0, "Command"="REFL{WfmSuffix}:REL:MIDD", "Access"=2, "Range Table"="RsScope_rngUserReferenceRelativeLevel", "Read Callback"="", "Write Callback"="", "Supported Models"="", "Instrument Options"="", "Flags"=0, "Help"="Sets the middle relative reference level, defined as a percentage of the high signal level.\n\nNote:\nRequires RSSCOPE_ATTR_REFERENCE_LEVEL_RELATIVE_LEVELS to be set to USER.\n\nAvailable Repeated Capabilities:\nWfmSuffix: WfmNone, WfmC1W1, WfmC1W2, WfmC1W3, WfmC2W1, WfmC2W2, WfmC2W3, WfmC3W1, WfmC3W2, WfmC3W3, WfmC4W1, WfmC4W2, WfmC4W3, WfmMath1, WfmMath2, WfmMath3, WfmMath4, WfmRef1, WfmRef2, WfmRef3, WfmRef4, WfmXY1, WfmXY2, WfmXY3, WfmXY4, WfmMeas1, WfmMeas2, WfmMeas3, WfmMeas4, WfmMeas5, WfmMeas6, WfmMeas7, WfmMeas8, WfmSbus1, WfmSbus2, WfmSbus3, WfmSbus4, WfmD0, WfmD1, WfmD2, WfmD3, WfmD4, WfmD5, WfmD6, WfmD7, WfmD8, WfmD9, WfmD10, WfmD11, WfmD12, WfmD13, WfmD14, WfmD15, WfmMSO1, WfmMSO2, WfmMSO3, WfmMSO4, WfmTRK1, WfmTRK2, WfmTRK3, WfmTRK4, WfmTRK5, WfmTRK6, WfmTRK7, WfmTRK8, WfmSpectrum1, WfmSpectrum2, WfmSpectrum3, WfmSpectrum4, WfmSG1TL1, WfmSG1TL2, WfmSG2TL1, WfmSG2TL2, WfmSG3TL1, WfmSG3TL2, WfmSG4TL1, WfmSG4TL2, WfmEye1, WfmEye2, WfmEye3, WfmEye4, WfmZ1V1, WfmZ1V2, WfmZ1V3, WfmZ1V4, WfmZ1I1, WfmZ1I2, WfmZ1I3, WfmZ1I4, WfmZ2V1, WfmZ2V2, WfmZ2V3, WfmZ2V4, WfmZ2I1, WfmZ2I2, WfmZ2I3, WfmZ2I4, WfmDiff1, WfmDiff2, WfmCommon1, WfmCommon2, WfmTDRZ, WfmTDRH, WfmTDRR, WfmMath5, WfmMath6, WfmMath7, WfmMath8, WfmSpectrum5, WfmSpectrum6, WfmSpectrum7, WfmSpectrum8, WfmSG5TL1, WfmSG5TL2, WfmSG6TL1, WfmSG6TL2, WfmSG7TL1, WfmSG7TL2, WfmSG8TL1, WfmSG8TL2, WfmHP1, WfmHP2, WfmHP3, WfmHP4, WfmHP5, WfmHP6, WfmHP7, WfmHP8, WfmHP9, WfmHP10, WfmBathtub1, WfmBathMeas1, WfmStepResp1, WfmSRHist1, WfmSDHist1, WfmTJHist1, WfmDJHist1, WfmDDJHist1, WfmPJHist1, WfmRJOHist1, WfmSRTrack1, WfmTJTrack1, WfmDJTrack1, WfmDDJTrack1, WfmPJTrack1, WfmRJTrack1, WfmTJSpectrum1, WfmDDJSpectrum1, WfmPJSpectrum1, WfmRJSpectrum1, WfmSEye1, WfmBathtub2, WfmBathMeas2, WfmStepResp2, WfmSRHist2, WfmSDHist2, WfmTJHist2, WfmDJHist2, WfmDDJHist2, WfmPJHist2, WfmRJOHist2, WfmSRTrack2, WfmSDTrack2, WfmTJTrack2, WfmDDJTrack2, WfmPJTrack2, WfmRJTrack2, WfmTJSpectrum2, WfmDDJSpectrum2, WfmPJSpectrum2, WfmRJSpectrum2, WfmSEye2, WfmNBathtub1, WfmNBathMeas1, WfmTNHist1, WfmDNHist1, WfmDDNHist1, WfmPNHist1, WfmRNOTrack1, WfmTNTrack1, WfmDDNTrack1, WfmPNTrack1, WfmRNTrack1, WfmTNSpectrum1, WfmDDNSpectrum1, WfmPNSpectrum1, WfmRNSpectrum1, WfmNBathtub2, WfmNBathMeas2, WfmTNHist2, WfmDNHist2, WfmDDNHist2, WfmPNHist2, WfmRNOHist2, WfmTNTrack2, WfmDDNTrack2, WfmPNTrack2, WfmRNTrack2, WfmTNSpectrum2, WfmDDNSpectrum2, WfmPNSpectrum2, WfmRNSpectrum2, WfmPJDHist1, WfmBUJHist1, WfmRJHist1, WfmPJDTrack1, WfmPJDSpectrum1, WfmPJDHist2, WfmBUJHist2, WfmRJHist2, WfmPJDTrack2, WfmPJDSpectrum2, WfmPNDHist1, WfmBUNHist1, WfmRNHist1, WfmPNDTrack1, WfmPNDSpectrum1, WfmPNDHist2, WfmBUNHist2, WfmRNHist2, WfmPNDTrack2, WfmPNDSpectrum2\r\n\nRemote-control command(s):\nREFLevel<m>:RELative:MIDDle"}, {"Level"=3, "Class Only"=FALSE, "Identifier"="RSSCOPE_ATTR_USER_REFERENCE_RELATIVE_LOWER_LEVEL", "Descriptive Name"="User Reference Relative Lower Level", "Data Type"=0, "Command"="REFL{WfmSuffix}:REL:LOW", "Access"=2, "Range Table"="RsScope_rngUserReferenceRelativeLevel", "Read Callback"="", "Write Callback"="", "Supported Models"="", "Instrument Options"="", "Flags"=0, "Help"="Sets the lower relative reference level, defined as a percentage of the high signal level.\n\nNote:\nRequires RSSCOPE_ATTR_REFERENCE_LEVEL_RELATIVE_LEVELS to be set to USER.\n\nAvailable Repeated Capabilities:\nWfmSuffix: WfmNone, WfmC1W1, WfmC1W2, WfmC1W3, WfmC2W1, WfmC2W2, WfmC2W3, WfmC3W1, WfmC3W2, WfmC3W3, WfmC4W1, WfmC4W2, WfmC4W3, WfmMath1, WfmMath2, WfmMath3, WfmMath4, WfmRef1, WfmRef2, WfmRef3, WfmRef4, WfmXY1, WfmXY2, WfmXY3, WfmXY4, WfmMeas1, WfmMeas2, WfmMeas3, WfmMeas4, WfmMeas5, WfmMeas6, WfmMeas7, WfmMeas8, WfmSbus1, WfmSbus2, WfmSbus3, WfmSbus4, WfmD0, WfmD1, WfmD2, WfmD3, WfmD4, WfmD5, WfmD6, WfmD7, WfmD8, WfmD9, WfmD10, WfmD11, WfmD12, WfmD13, WfmD14, WfmD15, WfmMSO1, WfmMSO2, WfmMSO3, WfmMSO4, WfmTRK1, WfmTRK2, WfmTRK3, WfmTRK4, WfmTRK5, WfmTRK6, WfmTRK7, WfmTRK8, WfmSpectrum1, WfmSpectrum2, WfmSpectrum3, WfmSpectrum4, WfmSG1TL1, WfmSG1TL2, WfmSG2TL1, WfmSG2TL2, WfmSG3TL1, WfmSG3TL2, WfmSG4TL1, WfmSG4TL2, WfmEye1, WfmEye2, WfmEye3, WfmEye4, WfmZ1V1, WfmZ1V2, WfmZ1V3, WfmZ1V4, WfmZ1I1, WfmZ1I2, WfmZ1I3, WfmZ1I4, WfmZ2V1, WfmZ2V2, WfmZ2V3, WfmZ2V4, WfmZ2I1, WfmZ2I2, WfmZ2I3, WfmZ2I4, WfmDiff1, WfmDiff2, WfmCommon1, WfmCommon2, WfmTDRZ, WfmTDRH, WfmTDRR, WfmMath5, WfmMath6, WfmMath7, WfmMath8, WfmSpectrum5, WfmSpectrum6, WfmSpectrum7, WfmSpectrum8, WfmSG5TL1, WfmSG5TL2, WfmSG6TL1, WfmSG6TL2, WfmSG7TL1, WfmSG7TL2, WfmSG8TL1, WfmSG8TL2, WfmHP1, WfmHP2, WfmHP3, WfmHP4, WfmHP5, WfmHP6, WfmHP7, WfmHP8, WfmHP9, WfmHP10, WfmBathtub1, WfmBathMeas1, WfmStepResp1, WfmSRHist1, WfmSDHist1, WfmTJHist1, WfmDJHist1, WfmDDJHist1, WfmPJHist1, WfmRJOHist1, WfmSRTrack1, WfmTJTrack1, WfmDJTrack1, WfmDDJTrack1, WfmPJTrack1, WfmRJTrack1, WfmTJSpectrum1, WfmDDJSpectrum1, WfmPJSpectrum1, WfmRJSpectrum1, WfmSEye1, WfmBathtub2, WfmBathMeas2, WfmStepResp2, WfmSRHist2, WfmSDHist2, WfmTJHist2, WfmDJHist2, WfmDDJHist2, WfmPJHist2, WfmRJOHist2, WfmSRTrack2, WfmSDTrack2, WfmTJTrack2, WfmDDJTrack2, WfmPJTrack2, WfmRJTrack2, WfmTJSpectrum2, WfmDDJSpectrum2, WfmPJSpectrum2, WfmRJSpectrum2, WfmSEye2, WfmNBathtub1, WfmNBathMeas1, WfmTNHist1, WfmDNHist1, WfmDDNHist1, WfmPNHist1, WfmRNOTrack1, WfmTNTrack1, WfmDDNTrack1, WfmPNTrack1, WfmRNTrack1, WfmTNSpectrum1, WfmDDNSpectrum1, WfmPNSpectrum1, WfmRNSpectrum1, WfmNBathtub2, WfmNBathMeas2, WfmTNHist2, WfmDNHist2, WfmDDNHist2, WfmPNHist2, WfmRNOHist2, WfmTNTrack2, WfmDDNTrack2, WfmPNTrack2, WfmRNTrack2, WfmTNSpectrum2, WfmDDNSpectrum2, WfmPNSpectrum2, WfmRNSpectrum2, WfmPJDHist1, WfmBUJHist1, WfmRJHist1, WfmPJDTrack1, WfmPJDSpectrum1, WfmPJDHist2, WfmBUJHist2, WfmRJHist2, WfmPJDTrack2, WfmPJDSpectrum2, WfmPNDHist1, WfmBUNHist1, WfmRNHist1, WfmPNDTrack1, WfmPNDSpectrum1, WfmPNDHist2, WfmBUNHist2, WfmRNHist2, WfmPNDTrack2, WfmPNDSpectrum2\r\n\nRemote-control command(s):\nREFLevel<m>:RELative:LOWer"}, {"Level"=3, "Class Only"=FALSE, "Identifier"="RSSCOPE_ATTR_USER_REFERENCE_HYSTERESIS", "Descriptive Name"="User Reference Hysteresis", "Data Type"=1, "Command"="REFL{WfmSuffix}:REL:HYST", "Access"=2, "Range Table"="rsscope_rngHysteresis", "Read Callback"="", "Write Callback"="", "Supported Models"="", "Instrument Options"="", "Flags"=0, "Help"="Defines a hysteresis for the middle reference level. A rise or fall from the middle reference value that does not exceed the hysteresis is rejected as noise.\n\nAvailable Repeated Capabilities:\nWfmSuffix: WfmNone, WfmC1W1, WfmC1W2, WfmC1W3, WfmC2W1, WfmC2W2, WfmC2W3, WfmC3W1, WfmC3W2, WfmC3W3, WfmC4W1, WfmC4W2, WfmC4W3, WfmMath1, WfmMath2, WfmMath3, WfmMath4, WfmRef1, WfmRef2, WfmRef3, WfmRef4, WfmXY1, WfmXY2, WfmXY3, WfmXY4, WfmMeas1, WfmMeas2, WfmMeas3, WfmMeas4, WfmMeas5, WfmMeas6, WfmMeas7, WfmMeas8, WfmSbus1, WfmSbus2, WfmSbus3, WfmSbus4, WfmD0, WfmD1, WfmD2, WfmD3, WfmD4, WfmD5, WfmD6, WfmD7, WfmD8, WfmD9, WfmD10, WfmD11, WfmD12, WfmD13, WfmD14, WfmD15, WfmMSO1, WfmMSO2, WfmMSO3, WfmMSO4, WfmTRK1, WfmTRK2, WfmTRK3, WfmTRK4, WfmTRK5, WfmTRK6, WfmTRK7, WfmTRK8, WfmSpectrum1, WfmSpectrum2, WfmSpectrum3, WfmSpectrum4, WfmSG1TL1, WfmSG1TL2, WfmSG2TL1, WfmSG2TL2, WfmSG3TL1, WfmSG3TL2, WfmSG4TL1, WfmSG4TL2, WfmEye1, WfmEye2, WfmEye3, WfmEye4, WfmZ1V1, WfmZ1V2, WfmZ1V3, WfmZ1V4, WfmZ1I1, WfmZ1I2, WfmZ1I3, WfmZ1I4, WfmZ2V1, WfmZ2V2, WfmZ2V3, WfmZ2V4, WfmZ2I1, WfmZ2I2, WfmZ2I3, WfmZ2I4, WfmDiff1, WfmDiff2, WfmCommon1, WfmCommon2, WfmTDRZ, WfmTDRH, WfmTDRR, WfmMath5, WfmMath6, WfmMath7, WfmMath8, WfmSpectrum5, WfmSpectrum6, WfmSpectrum7, WfmSpectrum8, WfmSG5TL1, WfmSG5TL2, WfmSG6TL1, WfmSG6TL2, WfmSG7TL1, WfmSG7TL2, WfmSG8TL1, WfmSG8TL2, WfmHP1, WfmHP2, WfmHP3, WfmHP4, WfmHP5, WfmHP6, WfmHP7, WfmHP8, WfmHP9, WfmHP10, WfmBathtub1, WfmBathMeas1, WfmStepResp1, WfmSRHist1, WfmSDHist1, WfmTJHist1, WfmDJHist1, WfmDDJHist1, WfmPJHist1, WfmRJOHist1, WfmSRTrack1, WfmTJTrack1, WfmDJTrack1, WfmDDJTrack1, WfmPJTrack1, WfmRJTrack1, WfmTJSpectrum1, WfmDDJSpectrum1, WfmPJSpectrum1, WfmRJSpectrum1, WfmSEye1, WfmBathtub2, WfmBathMeas2, WfmStepResp2, WfmSRHist2, WfmSDHist2, WfmTJHist2, WfmDJHist2, WfmDDJHist2, WfmPJHist2, WfmRJOHist2, WfmSRTrack2, WfmSDTrack2, WfmTJTrack2, WfmDDJTrack2, WfmPJTrack2, WfmRJTrack2, WfmTJSpectrum2, WfmDDJSpectrum2, WfmPJSpectrum2, WfmRJSpectrum2, WfmSEye2, WfmNBathtub1, WfmNBathMeas1, WfmTNHist1, WfmDNHist1, WfmDDNHist1, WfmPNHist1, WfmRNOTrack1, WfmTNTrack1, WfmDDNTrack1, WfmPNTrack1, WfmRNTrack1, WfmTNSpectrum1, 
